vi "encoderQueue.vi"(8 "error in (no error)":errorcluster, 11 "Command":T1) -> (0 "error out":errorcluster, 3 "queue out":refnum<queue>)   [LabVIEW 2017, in "externalAquisition.lvlib"]
uses:
  externalAquisition.lvlib
  TypeDefs/QueueCommands.ctl
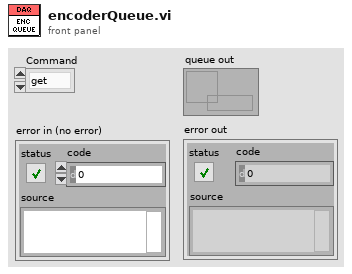
[diagram p1: front panel]
types:
  T1 = typedef "externalAquisition.lvlib/QueueCommands.ctl" = enum16{"get", "set"}
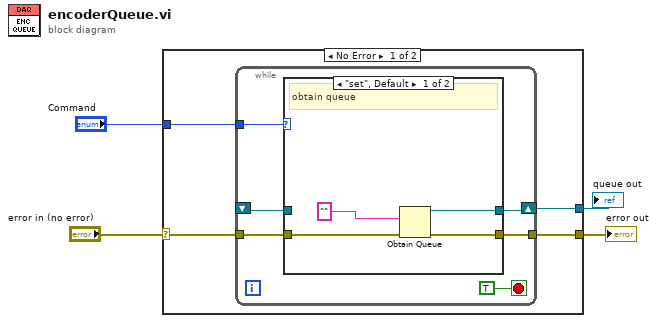
[diagram p0: block diagram]
diagram:
  n1 = case shown="No Error" "error in (no error)" {
    selector: "error in (no error)" -> [w7 w21]
    tunnel: [w6 w21] -> w3
    tunnel: "Command" -> [w8 _]
    tunnel: [w5 _] -> w1
    frame No Error {
      n2 = while {
        tunnel: w8 -> [w13]
        tunnel: w7 -> [w12]
        tunnel: [w11] -> w6
        shift-right: [w10] -> w5
        shift-left: _ -> [w9]
        stop <- TRUE stop-if-true
        n3 = case shown="\"set\", Default" w13 {
          tunnel: w12 -> [w18 w20]
          tunnel: [w17 w20] -> w11
          tunnel: [w16 w19] -> w10
          tunnel: w9 -> [_ w19]
          frame "set", Default {
            # "obtain queue"
            n4 = Obtain Queue(element data type="", error in (no error)=w18) -> (queue out=w16:refnum<queue>, error out=w17:errorcluster)  [unwired: 3 in, 1 out]
          }
          frame "get" {
            # "get queue ref"
          }
        }
      }
    }
    frame Error {
    }
  }
  "error out" <- w3
  "queue out" <- w1
